vi "m1m3_getEvent_AirSupplyWarning.vi"(8 "error in (no error)":errorcluster, 11 "logevent_AirSupplyWarning_Ctl":T1) -> (0 "error out":errorcluster, 2 "function return":i32, 3 "logevent_AirSupplyWarning_Ctl out":T1)   [LabVIEW 2016, in "SALLV_m1m3.lvlib"]
doc: "int m1m3_shm_getEvent_AirSupplyWarningLV(m1m3_logevent_AirSupplyWarningLV *logevent_AirSupplyWarning_Ctl );"
uses:
  SALLV_m1m3.lvlib
  DataTypes/logevent_AirSupplyWarning.ctl
  SALLV_m1m3.so
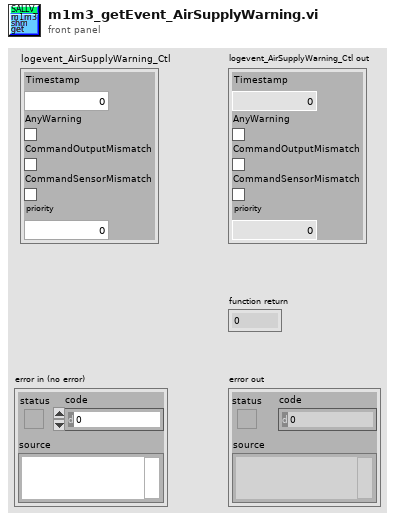
[diagram p1: front panel]
types:
  T1 = typedef "SALLV_m1m3.lvlib/logevent_AirSupplyWarning.ctl" = cluster{"Timestamp":dbl, "AnyWarning":bool, "CommandOutputMismatch":bool, "CommandSensorMismatch":bool, "priority":i32}
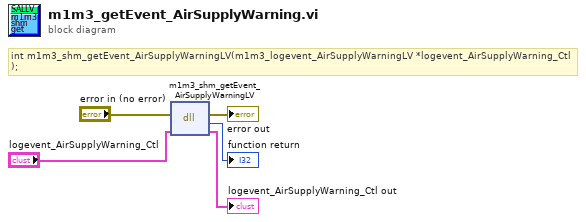
[diagram p0: block diagram]
diagram:
  # "int m1m3_shm_getEvent_AirSupplyWarningLV(m1m3_logevent_AirSupplyWarningLV *logevent_AirSupplyWarning_Ctl );"
  n1 = dll-call lib="opt/CODE/SALLV_m1m3/SALLV_m1m3.*" fn="m1m3_shm_getEvent_AirSupplyWarningLV"(error in="error in (no error)", "logevent_AirSupplyWarning_Ctl"="logevent_AirSupplyWarning_Ctl") -> (error out=→"error out":errorcluster, →"function return":i32, "logevent_AirSupplyWarning_Ctl"=→"logevent_AirSupplyWarning_Ctl out":T1)  [unwired: 2 in, 1 out]
